vi "Process.vi"(8 "error in (no error)":errorcluster, 11 "ConfigManager.Text in":refnum<class "ConfigManager.Text.lvclass">) -> (0 "error out":errorcluster, 3 "ConfigManager.Text out":refnum<class "ConfigManager.Text.lvclass">)   [LabVIEW 2013, in "CfgManager.Text.lvlib" / "ConfigManager.Text.lvclass"]
uses:
  ConfigManager.Text.lvclass
  ConfigManager.Text.lvclass/ConfigManager.Text.ctl
  Query -- cluster.ctl
  Response - cluster.ctl
  Update -- cluster.ctl
  Dictionary Payload -- cluster.ctl
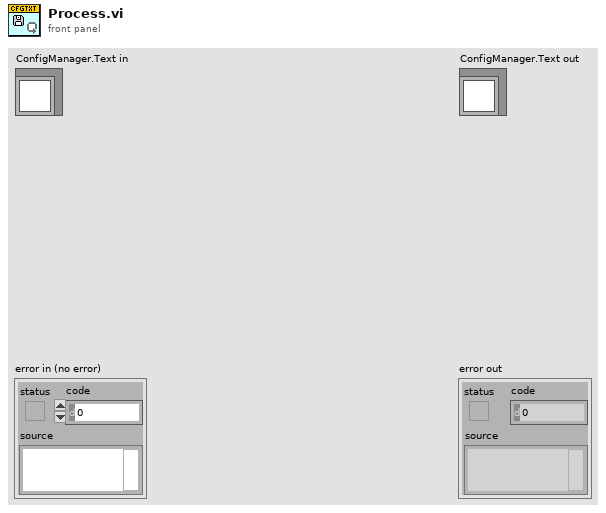
[diagram p1: front panel]
types:
  T1 = typedef "CfgManager.Text.lvlib/ConfigManager.Text.lvclass/Response - cluster.ctl" = cluster{"Section":string[], "Keys":string[], "Values":string[], "Found":bool[]}
  T2 = typedef "CfgManager.Text.lvlib/ConfigManager.Text.lvclass/Dictionary Payload -- cluster.ctl" = cluster{"Value":string, "Comment":string, "stack position":i32}
  T3 = typedef "CfgManager.Text.lvlib/ConfigManager.Text.lvclass/payload -- cluster.ctl" = cluster{"command":string, "args":variant, "query":refnum<notifier>, "ack":refnum<notifier>}
  T4 = typedef "CfgManager.Text.lvlib/ConfigManager.Text.lvclass/Query -- cluster.ctl" = cluster{"Qualified Name":string[], "Keys":string[]}
  T5 = typedef "CfgManager.Text.lvlib/ConfigManager.Text.lvclass/Update -- cluster.ctl" = cluster{"Qualified Name":string[], "Keys":string[], "Values":string[]}
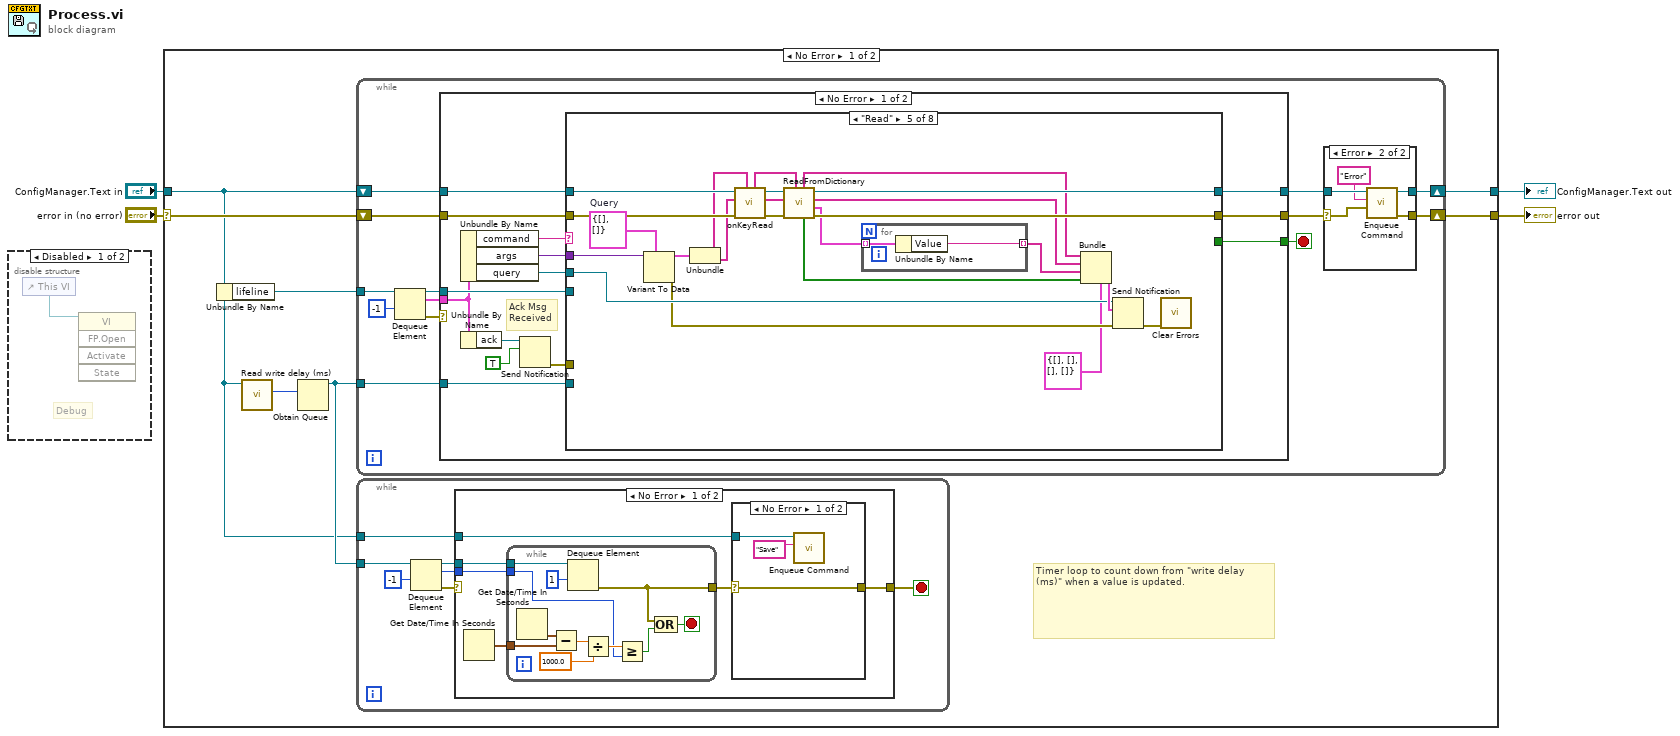
[diagram p0: block diagram]
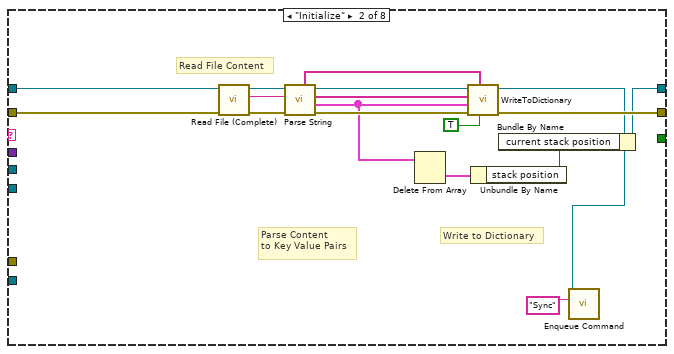
[diagram p7: hidden frame]
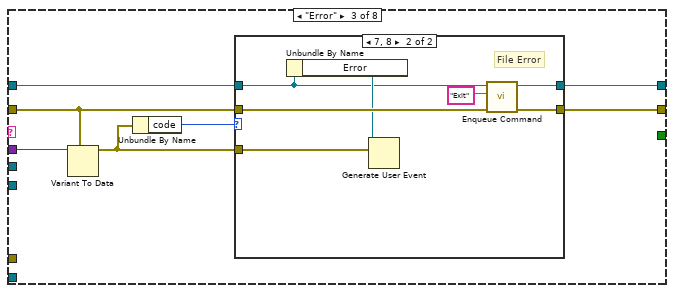
[diagram p8: hidden frame]
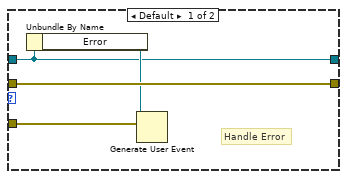
[diagram p9: hidden frame]
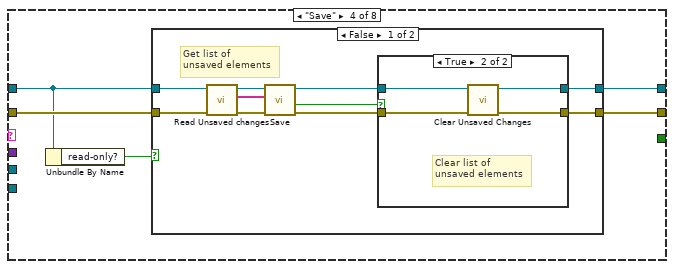
[diagram p10: hidden frame]
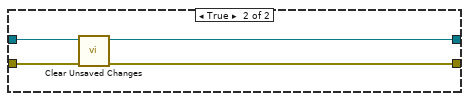
[diagram p12: hidden frame]
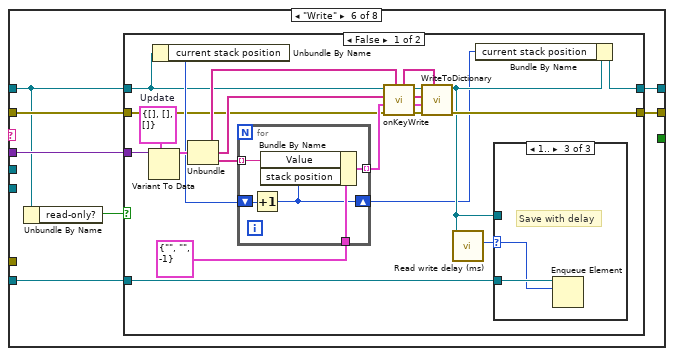
[diagram p13: hidden frame]
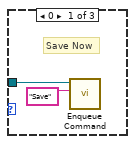
[diagram p14: hidden frame]
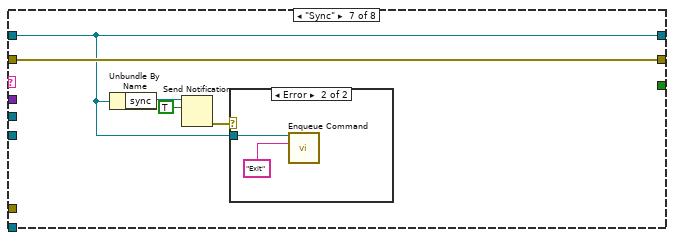
[diagram p17: hidden frame]
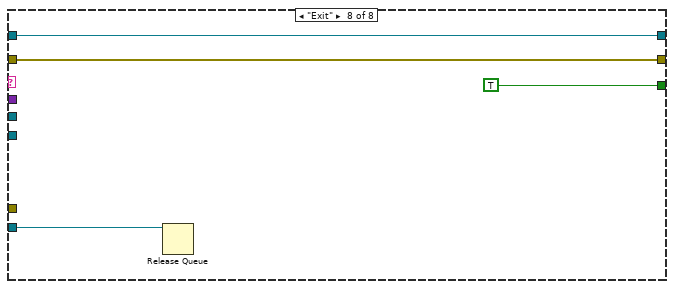
[diagram p19: hidden frame]
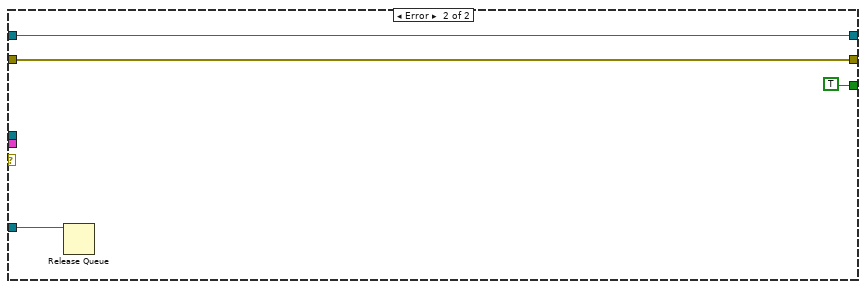
[diagram p20: hidden frame]
diagram:
  n1 = disable-structure shown="Disabled" {
    frame Disabled {
      # "Debug"
      n2 = control-ref of="This VI"() -> (w5:refnum<vi>)
      n3 = invoke class="VI" method="FP.Open"(reference=w5) -> ()  [unwired: 4 in, 5 out]
    }
    frame Enabled {
    }
  }
  n4 = case shown="No Error" "error in (no error)" {
    selector: "error in (no error)" -> [w12 w216]
    tunnel: [w10 w216] -> w3
    tunnel: [w11 w215] -> w1
    tunnel: "ConfigManager.Text in" -> [w7 w215]
    frame No Error {
      # "Timer loop to count down from \"write delay (ms)\" when a value is updated."
      n5 = Unbundle By Name(w7) -> ("lifeline"=w8:refnum<queue>)
      n6 = call "Read write delay (ms).vi"("ConfigManager.Text in"=w7) -> ("write delay (ms)"=w6:i32)  [unwired: 9 in, 1 out]
      n7 = Obtain Queue(element data type=w6) -> (queue out=w9:refnum<queue>)  [unwired: 4 in, 2 out]
      n8 = while {
        shift-right: [w44] -> w11
        shift-left: w7 -> [w54]
        tunnel: w8 -> [w51]
        tunnel: w9 -> [w46]
        shift-right: [w42] -> w10
        shift-left: w12 -> [w53]
        stop <- w49 stop-if-true
        n9 = Dequeue Element(queue=w51, timeout in ms (-1)=-1) -> (queue out=w47:refnum<queue>, element=w48:T3, error out=w50:errorcluster)  [unwired: 1 in, 1 out]
        n10 = case shown="No Error" w50 {
          tunnel: w54 -> [w75 w213]
          tunnel: [w72 w213] -> w45
          tunnel: w53 -> [w73 w212]
          tunnel: [w71 w212] -> w43
          tunnel: [w69 TRUE] -> w49
          tunnel: w48 -> [w66 _]
          tunnel: w47 -> [w68 _]
          tunnel: w46 -> [w62 w211]
          frame No Error {
            # "Ack Msg\nReceived"
            n11 = Unbundle By Name(w66) -> ("command"=w74:string, "args"=w70:variant, "query"=w67:refnum<notifier>)
            n12 = Unbundle By Name(w66) -> ("ack"=w65:refnum<notifier>)
            n13 = Send Notification(notification=TRUE, notifier=w65) -> (error out=w63:errorcluster)  [unwired: 1 in, 1 out]
            n14 = case shown="\"Read\"" w74 {
              tunnel: w75 -> [w77 w85 w96 w114 w142 w162 w200 w208]
              tunnel: w73 -> [w76 w79 w98 w117 w140 w164 w204 w207]
              tunnel: [w77 w81 w101 w116 w157 w161 w200 w208] -> w72
              tunnel: [w76 w92 w100 w115 w156 w165 w204 w207] -> w71
              tunnel: w70 -> [_ _ w99 _ w153 w166 _ _]
              tunnel: [_ _ _ _ _ _ _ TRUE] -> w69
              tunnel: w68 -> [_ _ _ _ _ _ _ _]
              tunnel: w67 -> [_ _ _ _ w152 _ _ _]
              tunnel: w63 -> [_ _ _ _ _ _ _ _]
              tunnel: w62 -> [_ _ _ _ _ w163 _ w209]
              frame Default {
              }
              frame "Initialize" {
                # "Write to Dictionary"
                # "Parse Content\nto Key Value Pairs"
                # "Read File Content"
                n15 = call "Read File (Complete).vi"("error in (no error)"=w79, "ConfigManager.Text in"=w85) -> ("error out"=w89:errorcluster, "String"=w90:string, "ConfigManager.Text out"=w91:refnum<class "ConfigManager.Text.lvclass">)  [unwired: 7 in]
                n16 = call-dynamic "Parse String.vi"("error in (no error)"=w89, "Input String"=w90, "ConfigManager.Text in"=w91) -> ("error out"=w93:errorcluster, "Content"=w83:T2[], "Keys"=w94:string[], "ConfigManager.Text out"=w88:refnum<class "ConfigManager.Text.lvclass">, "Section"=w86:string[])  [unwired: 4 in]
                n17 = Delete From Array(array=w83) -> (deleted portion=w82:T2)  [unwired: 2 in, 1 out]
                n18 = call "WriteToDictionary.vi"("Initial call"=TRUE, "Section"=w86, "error in (no error)"=w93, "Content"=w83, "Keys"=w94, "ConfigManager.Text in"=w88) -> ("error out"=w92:errorcluster, "ConfigManager.Text out"=w78:refnum<class "ConfigManager.Text.lvclass">)  [unwired: 4 in]
                n19 = Unbundle By Name(w82) -> ("stack position"=w80:i32)
                n20 = Bundle By Name(cluster=w78, "current stack position"=w80) -> (w81:refnum<class "ConfigManager.Text.lvclass">)
                n21 = call "Enqueue Command.vi"("command"="Sync", "ConfigManager.Text in"=w78) -> ()  [unwired: 7 in, 3 out]
              }
              frame "Error" {
                n22 = Variant To Data(type=w98, Variant=w99) -> (data=w95:errorcluster)  [unwired: 1 in, 1 out]
                n23 = Unbundle By Name(w95) -> ("code"=w97:i32)
                n24 = case shown="7, 8" w97 {
                  tunnel: w96 -> [w103 w107]
                  tunnel: [w103 w111] -> w101
                  tunnel: [w105 w110] -> w100
                  tunnel: w98 -> [w105 w109]
                  tunnel: w95 -> [w102 w106]
                  frame Default {
                    # "Handle Error"
                    n25 = Unbundle By Name(w103) -> ("Error"=w104:refnum<user-event>)
                    n26 = Generate User Event(user event=w104, event data cluster=w102) -> ()  [unwired: 2 in, 2 out]
                  }
                  frame 7, 8 {
                    # "File Error"
                    n27 = Unbundle By Name(w107) -> ("Error"=w108:refnum<user-event>)
                    n28 = Generate User Event(user event=w108, event data cluster=w106) -> ()  [unwired: 2 in, 2 out]
                    n29 = call "Enqueue Command.vi"("error in (no error)"=w109, "command"="Exit", "ConfigManager.Text in"=w107) -> ("error out"=w110:errorcluster, "ConfigManager.Text out"=w111:refnum<class "ConfigManager.Text.lvclass">)  [unwired: 6 in, 1 out]
                  }
                }
              }
              frame "Save" {
                n30 = Unbundle By Name(w114) -> ("read-only?"=w113:bool)
                n31 = case shown="False" w113 {
                  tunnel: w117 -> [w126 w132]
                  tunnel: [w122 w133] -> w116
                  tunnel: [w119 w132] -> w115
                  tunnel: w114 -> [w118 w134]
                  frame False {
                    # "Get list of\nunsaved elements"
                    n32 = call "Read Unsaved changes.vi"("ConfigManager.Text in"=w118) -> ("Unsaved changes"=w125:string[], "ConfigManager.Text out"=w124:refnum<class "ConfigManager.Text.lvclass">)  [unwired: 9 in]
                    n33 = call-dynamic "Save.vi"("error in (no error)"=w126, "Elements changed"=w125, "ConfigManager.Text in"=w124) -> ("error out"=w120:errorcluster, "success"=w121:bool, "ConfigManager.Text out"=w123:refnum<class "ConfigManager.Text.lvclass">)  [unwired: 6 in]
                    n34 = case shown="True" w121 {
                      tunnel: w123 -> [w127 w131]
                      tunnel: [w127 w130] -> w122
                      tunnel: w120 -> [w128 w129]
                      tunnel: [w128 w129] -> w119
                      frame False {
                      }
                      frame True {
                        # "Clear list of\nunsaved elements"
                        n35 = call "Clear Unsaved Changes.vi"("ConfigManager.Text in"=w131) -> ("ConfigManager.Text out"=w130:refnum<class "ConfigManager.Text.lvclass">)  [unwired: 10 in]
                      }
                    }
                  }
                  frame True {
                    n36 = call "Clear Unsaved Changes.vi"("ConfigManager.Text in"=w134) -> ("ConfigManager.Text out"=w133:refnum<class "ConfigManager.Text.lvclass">)  [unwired: 10 in]
                  }
                }
              }
              frame "Read" {
                w149 = T4 {"Qualified Name"=[], "Keys"=[]}  # Query
                n37 = Variant To Data(type=w149, Variant=w153) -> (data=w148:T4, error out=w151:errorcluster)  [unwired: 1 in]
                n38 = Unbundle(w148) -> ("Qualified Name"=w138:string[], "Keys"=w137:string[])
                n39 = call-dynamic "onKeyRead.vi"("Qualified Name"=w138, "error in (no error)"=w140, "Keys"=w137, "ConfigManager.Text in"=w142) -> ("error out"=w139:errorcluster, "Keys out"=w136:string[], "ConfigManager.Text out"=w141:refnum<class "ConfigManager.Text.lvclass">, "Qualified Name out"=w135:string[])  [unwired: 4 in]
                n40 = call "ReadFromDictionary.vi"("Section"=w135, "error in (no error)"=w139, "Keys"=w136, "ConfigManager.Text in"=w141) -> ("error out"=w156:errorcluster, "Content"=w144:T2[], "Keys out"=w155:string[], "ConfigManager.Text out"=w157:refnum<class "ConfigManager.Text.lvclass">, "Found"=w146:bool[], "Section"=w145:string[])  [unwired: 2 in]
                n41 = for {
                  tunnel: w144 -> [w159] mode=indexing
                  tunnel: [w158] -> w143 mode=indexing
                  n42 = Unbundle By Name(w159) -> ("Value"=w158:string)
                }
                n43 = Bundle(cluster=T1 {"Section"=[], "Keys"=[], "Values"=[], "Found"=[]} ("response"), "Section"=w145, "Keys"=w155, "Values"=w143, "Found"=w146) -> (w154:T1)
                n44 = Send Notification(notification=w154, notifier=w152, error in (no error)=w151) -> (error out=w150:errorcluster)  [unwired: 1 out]
                n45 = call <vilib>:"Clear Errors.vi"("error in (no error)"=w150) -> ()  [unwired: 6 in, 1 out]
              }
              frame "Write" {
                n46 = Unbundle By Name(w162) -> ("read-only?"=w160:bool)
                n47 = case shown="False" w160 {
                  tunnel: w166 -> [w188 _]
                  tunnel: [w185 w198] -> w165
                  tunnel: w164 -> [w168 w198]
                  tunnel: w163 -> [w184 _]
                  tunnel: w162 -> [w170 w199]
                  tunnel: [w179 w199] -> w161
                  frame False {
                    w186 = T5 {"Qualified Name"=[], "Keys"=[], "Values"=[]}  # Update
                    n48 = Variant To Data(type=w186, Variant=w188) -> (data=w187:T5)  [unwired: 1 in, 1 out]
                    n49 = Unbundle By Name(w170) -> ("current stack position"=w178:i32)
                    n50 = Unbundle(w187) -> ("Qualified Name"=w176:string[], "Keys"=w174:string[], "Values"=w181:string[])
                    n51 = for {
                      tunnel: T2 {"Value"="", "Comment"="", "stack position"=-1} ("Dictionary Payload") -> [w191]
                      tunnel: w181 -> [w193] mode=indexing
                      tunnel: [w192] -> w171 mode=indexing
                      shift-right: [w189] -> w177
                      shift-left: w178 -> [w190]
                      n52 = Increment(x=w190) -> (x+1=w189:i32)
                      n53 = Bundle By Name(cluster=w191, "Value"=w193, "stack position"=w189) -> (w192:T2)
                    }
                    n54 = call-dynamic "onKeyWrite.vi"("Qualified Name"=w176, "error in (no error)"=w168, "Content"=w171, "Keys"=w174, "ConfigManager.Text in"=w170) -> ("error out"=w167:errorcluster, "Content out"=w172:T2[], "Keys out"=w173:string[], "ConfigManager.Text out"=w169:refnum<class "ConfigManager.Text.lvclass">, "Qualified Name out"=w175:string[])  [unwired: 2 in]
                    n55 = call "WriteToDictionary.vi"("Section"=w175, "error in (no error)"=w167, "Content"=w172, "Keys"=w173, "ConfigManager.Text in"=w169) -> ("error out"=w185:errorcluster, "ConfigManager.Text out"=w180:refnum<class "ConfigManager.Text.lvclass">)  [unwired: 5 in]
                    n56 = call "Read write delay (ms).vi"("ConfigManager.Text in"=w180) -> ("write delay (ms)"=w183:i32)  [unwired: 9 in, 1 out]
                    n57 = Bundle By Name(cluster=w180, "current stack position"=w177) -> (w179:refnum<class "ConfigManager.Text.lvclass">)
                    n58 = case shown="1.." w183 {
                      selector: w183 -> [_ _ w196]
                      tunnel: w184 -> [_ _ w197]
                      tunnel: w180 -> [w195 _ _]
                      frame 0 {
                        # "Save Now"
                        n59 = call "Enqueue Command.vi"("command"="Save", "ConfigManager.Text in"=w195) -> ()  [unwired: 7 in, 3 out]
                      }
                      frame ..-1, Default {
                        # "Don't save"
                      }
                      frame 1.. {
                        # "Save with delay"
                        n60 = Enqueue Element(queue=w197, element=w196) -> ()  [unwired: 2 in, 3 out]
                      }
                    }
                  }
                  frame True {
                    # "Skip Write step for Read-Only files."
                  }
                }
              }
              frame "Sync" {
                n61 = Unbundle By Name(w200) -> ("sync"=w203:refnum<notifier>)
                n62 = Send Notification(notification=TRUE, notifier=w203) -> (error out=w201:errorcluster)  [unwired: 1 in, 1 out]
                n63 = case shown="Error" w201 {
                  tunnel: w200 -> [_ w206]
                  frame No Error {
                  }
                  frame Error {
                    n64 = call "Enqueue Command.vi"("command"="Exit", "ConfigManager.Text in"=w206) -> ()  [unwired: 7 in, 3 out]
                  }
                }
              }
              frame "Exit" {
                n65 = Release Queue(queue=w209) -> ()  [unwired: 2 in, 3 out]
              }
            }
          }
          frame Error {
            n66 = Release Queue(queue=w211) -> ()  [unwired: 2 in, 3 out]
          }
        }
        n67 = case shown="Error" w43 {
          selector: w43 -> [w55 w59]
          tunnel: w45 -> [w56 w61]
          tunnel: [w56 w60] -> w44
          tunnel: [w55 w57] -> w42
          frame No Error {
          }
          frame Error {
            n68 = call "Enqueue Command.vi"("args"=w59, "command"="Error", "ConfigManager.Text in"=w61) -> ("error out"=w57:errorcluster, "ConfigManager.Text out"=w60:refnum<class "ConfigManager.Text.lvclass">)  [unwired: 6 in, 1 out]
          }
        }
      }
      n69 = while {
        tunnel: w9 -> [w18]
        tunnel: w7 -> [w13]
        stop <- w16 stop-if-true
        n70 = Dequeue Element(queue=w18, timeout in ms (-1)=-1) -> (queue out=w14:refnum<queue>, element=w15:i32, error out=w17:errorcluster)  [unwired: 1 in, 1 out]
        n71 = case shown="No Error" w17 {
          selector: w17 -> [_ w41]
          tunnel: [w22 w41] -> w16
          tunnel: w15 -> [w25 _]
          tunnel: w14 -> [w24 _]
          tunnel: w13 -> [w21 _]
          frame No Error {
            n72 = Get Date/Time In Seconds() -> (seconds since 1Jan1904=w20:timestamp)
            n73 = while {
              tunnel: w25 -> [w31]
              tunnel: w24 -> [w40]
              tunnel: [w38] -> w23
              tunnel: w20 -> [w36]
              stop <- w37 stop-if-true
              n74 = Get Date/Time In Seconds() -> (seconds since 1Jan1904=w35:timestamp)
              n75 = Subtract(x=w35, y=w36) -> (x-y=w34:dbl)
              n76 = Dequeue Element(queue=w40, timeout in ms (-1)=1) -> (error out=w38:errorcluster)  [unwired: 1 in, 3 out]
              n77 = Divide(x=w34, y=1000.0) -> (x/y=w32:dbl)
              n78 = Greater Or Equal?(x=w32, y=w31) -> (x >= y?=w30:bool)
              n79 = Compound Arithmetic op=OR(w38, w30) -> (w37:bool)
            }
            n80 = case shown="No Error" w23 {
              selector: w23 -> [w28 w29]
              tunnel: [w28 w29] -> w22
              tunnel: w21 -> [w26 _]
              frame No Error {
                n81 = call "Enqueue Command.vi"("command"="Save", "ConfigManager.Text in"=w26) -> ()  [unwired: 7 in, 3 out]
              }
              frame Error {
              }
            }
          }
          frame Error {
          }
        }
      }
    }
    frame Error {
    }
  }
  "error out" <- w3
  "ConfigManager.Text out" <- w1
